vi "get_input_output_clusters.vi"(8 "error in":errorcluster, 9 "Input number":dbl, 10 "Output number":dbl, 11 "System cluster in":T2(array[cluster])) -> (0 "error out":errorcluster, 1 "Input element":T1, 2 "Output element":T1, 3 "System cluster out":T2(array[cluster]), 4 "index of output element":i32, 6 "index of input element":i32)   [LabVIEW 2010]
uses:
  <userlib>/_OpenG.lib/array/array.llb/Conditional Auto-Indexing Tunnel (Variant)__ogtk.vi
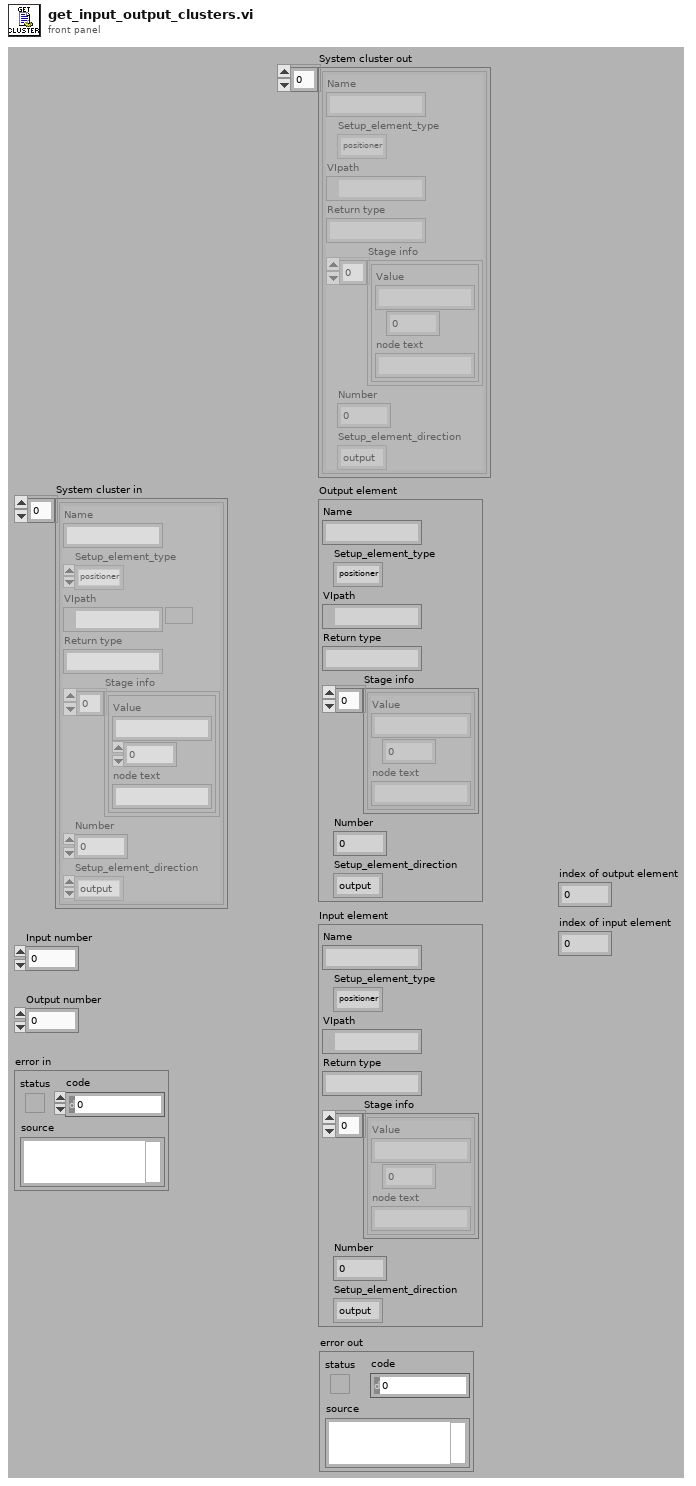
[diagram p1: front panel]
types:
  T1 = cluster{"Name":string, "Setup_element_type":enum16{"positioner", "acquisition", "synchronized"}, "VIpath":path, "Return type":string, "Stage info":cluster{"Value":string, i32, "node text":string}[], "Number":u32, "Setup_element_direction":enum16{"output", "input", "io"}}
  T2 = cluster{"Name":string, "Setup_element_type":enum16{"positioner", "acquisition", "synchronized"}, "VIpath":path, "Return type":string, "Stage info":cluster{"Value":string, i32, "node text":string}[], "Number":u32, "Setup_element_direction":enum16{"output", "input", "io"}}[]
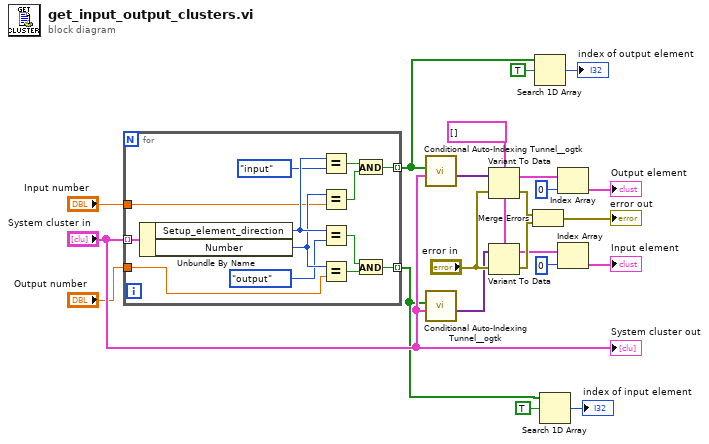
[diagram p0: block diagram]
diagram:
  w13 = T2 []
  n1 = for {
    tunnel: "System cluster in" -> [w35] mode=indexing
    tunnel: "Input number" -> [w30]
    tunnel: "Output number" -> [w29]
    tunnel: [w24] -> w6 mode=indexing
    tunnel: [w23] -> w1 mode=indexing
    n2 = Unbundle By Name(w35) -> ("Setup_element_direction"=w34:enum16{"output", "input", "io"}, "Number"=w33:u32)
    n3 = Equal?(x=w34, y=enum16{"output", "input", "io"}."input") -> (x = y?=w28:bool)
    n4 = Equal?(x=w33, y=w30) -> (x = y?=w27:bool)
    n5 = Equal?(x=w34, y=enum16{"output", "input", "io"}."output") -> (x = y?=w26:bool)
    n6 = Equal?(x=w33, y=w29) -> (x = y?=w25:bool)
    n7 = And(x=w28, y=w27) -> (x .and. y?=w24:bool)
    n8 = And(x=w26, y=w25) -> (x .and. y?=w23:bool)
  }
  n9 = call-poly <userlib>:"Conditional Auto-Indexing Tunnel__ogtk.vi"("Array in"="System cluster in", "Elements to keep"=w6) -> ("Filtered Array out"=w16:variant[])  [unwired: 5 in]
  n10 = call-poly <userlib>:"Conditional Auto-Indexing Tunnel__ogtk.vi"("Array in"="System cluster in", "Elements to keep"=w1) -> ("Filtered Array out"=w17:variant[])  [unwired: 5 in]
  n11 = Variant To Data(error in="error in", Variant=w16, type=w13) -> (error out=w19:errorcluster, data=w12:T2)
  n12 = Variant To Data(error in="error in", Variant=w17, type=w13) -> (error out=w20:errorcluster, data=w11:T2)
  n13 = Merge Errors(w19, w20) -> (→"error out":errorcluster)
  n14 = Search 1D Array(1D array=w6, element=TRUE) -> (index of element=→"index of output element":i32)  [unwired: 1 in]
  n15 = Search 1D Array(1D array=w1, element=TRUE) -> (index of element=→"index of input element":i32)  [unwired: 1 in]
  n16 = Index Array(array=w12, index=0) -> (element=→"Output element":T1)
  n17 = Index Array(array=w11, index=0) -> (element=→"Input element":T1)
  "System cluster out" <- "System cluster in"
